vi "Stop Core.vi"(10 "final error code":i32, 11 "Worker in":refnum<class "Worker.lvclass">) -> (3 "Worker out":refnum<class "Worker.lvclass">)   [LabVIEW 2023, in "Worker.lvlib" / "Worker.lvclass"]
doc: "(<B>Filename</B>: Actor Framework.lvlib:Actor.lvclass:Stop Core.vi)\n\nDefines what the actor does before it stops. Use the <B>final error code</B> input to determine whether the actor shut down in response to an error.\n\nBy default, this method does nothing. A descendant class may override it to define behavior, such as shutting down any processes the actor initiated in its override of the Actor Core method."
uses:
  Worker.lvclass
  Worker.lvclass/Worker.ctl
  Person/Person.lvclass
panel:
  out "error out":errorcluster
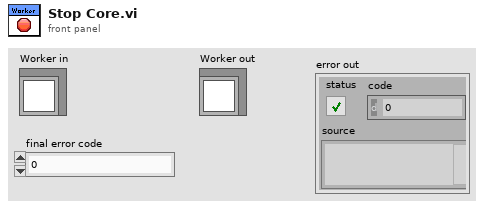
[diagram p1: front panel]
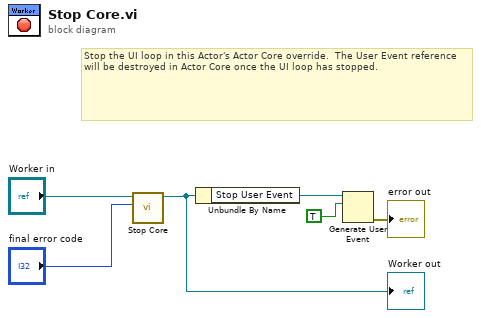
[diagram p0: block diagram]
diagram:
  # "Stop the UI loop in this Actor's Actor Core override.  The User Event reference will be destroyed in Actor Core once the UI loop has stopped."
  n1 = call-parent "Stop Core.vi"("final error code"="final error code", "Person in"="Worker in") -> ("Person out"=w2:refnum<class "Worker.lvclass">)  [unwired: 9 in]
  "Worker out" <- w2
  n2 = Unbundle By Name(w2) -> ("Stop User Event"=w4:refnum<user-event>)
  n3 = Generate User Event(user event=w4, event data cluster=TRUE ("event data")) -> (error out=→"error out":errorcluster)  [unwired: 2 in, 1 out]
